vi "Set Shifter.vi"(8 "error in (no error)":errorcluster, 11 "High Gear?":bool) -> (0 "error out":errorcluster)   [LabVIEW 2018]
uses:
  <vilib>/Rock Robotics/WPI/Solenoid/WPI_SolenoidValue.ctl
  Implementation/Is High Gear.vi
  <vilib>/Rock Robotics/WPI/Solenoid/WPI_SolenoidSetEnum.vi
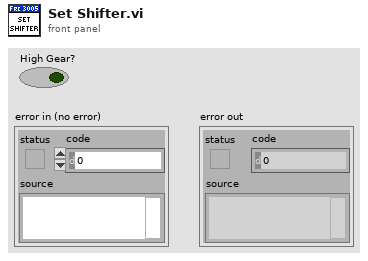
[diagram p1: front panel]
types:
  T1 = typedef "WPI_SolenoidValue.ctl" = enum16{"Off", "On", "Forward", "Reverse"}
  T2 = typedef "SPARKMAX6Motor.ctl" = cluster{"FrontLeftMaster":T3, "FrontLeftSlave1":T3, "FrontLeftSlave2":T3, "FrontRightMaster":T3, "FrontRightSlave1":T3, "FrontRightSlave2":T3}
  T3 = typedef "WPI_MotorControlDeviceRef.ctl" = cluster{"DeviceStatus":errorcluster, "Type":T4, "PWM":cluster{"PWM Channel":T5, "DeadBand":T6}, "CAN":cluster{"Device Number":u8, "SetOutput VI Ref":variant, "GetOutput VI Ref":variant, "Enable VI Ref":variant, "Disable VI Ref":variant, "Data":variant}, "Invert":bool, "DIO PWM":cluster{"PWM \"Enable\" Channel":T5, "DIOChannel":T7, "PWM Rate":dbl}}
  T4 = typedef "WPI_MotorControlType.ctl" = enum16{"PWM", "CAN", "DIO PWM"}
  T5 = typedef "FPGA_DIOPWMChannel.ctl" = enum8{"PWM 0", "PWM 1", "PWM 2", "PWM 3", "PWM 4", "PWM 5", "PWM 6", "PWM 7", "PWM 8", "PWM 9", "PWM MXP 0", "PWM MXP 1", "PWM MXP 2", "PWM MXP 3", "PWM MXP 4", "PWM MXP 5", "PWM MXP 6", "PWM MXP 7", "PWM MXP 8", "PWM MXP 9", "Invalid"}
  T6 = typedef "WPI_PWMDeadband.ctl" = cluster{"Name":string, "maxPositivePwm":i32, "minPositivePwm":i32, "centerPwm":i32, "maxNegativePwm":i32, "minNegativePwm":i32, "angularRange":u16}
  T7 = typedef "FPGA_DIOChannel.ctl" = enum8{"DIO 0", "DIO 1", "DIO 2", "DIO 3", "DIO 4", "DIO 5", "DIO 6", "DIO 7", "DIO 8", "DIO 9", "DIO MXP 0", "DIO MXP 1", "DIO MXP 2", "DIO MXP 3", "DIO MXP 4", "DIO MXP 5", "DIO MXP 6", "DIO MXP 7", "DIO MXP 8", "DIO MXP 9", "DIO MXP 10", "DIO MXP 11", "DIO MXP 12", "DIO MXP 13", "DIO MXP 14", "DIO MXP 15", "SPI Port CS1", "SPI Port CS2", "SPI Port CS3", "SPI Port MISO", "SPI Port MOSI", "Invalid"}
  T8 = typedef "WPI_SolenoidDevRef.ctl" = cluster{"DevStatus":errorcluster, "Pneumatics Control Module":u8, "Forward Solenoid Channel":T9, "Reverse Solenoid Channel":T9}
  T9 = typedef "WPI_SolenoidChannel.ctl" = enum8{"Solenoid 0", "Solenoid 1", "Solenoid 2", "Solenoid 3", "Solenoid 4", "Solenoid 5", "Solenoid 6", "Solenoid 7", "Invalid"}
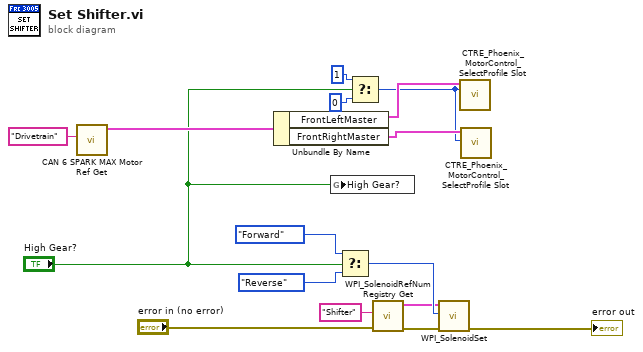
[diagram p0: block diagram]
diagram:
  n1 = call "CAN 6 SPARK MAX Motor Ref Get.vi"("refnum name"="Drivetrain") -> ("TalonSRX6MotorRef out"=w7:T2)  [unwired: 9 in, 1 out]
  n2 = Unbundle By Name(w7) -> ("FrontLeftMaster"=w6:T3, "FrontRightMaster"=w3:T3)
  n3 = global write "Is High Gear.vi" "High Gear?"("High Gear?") -> ()
  n4 = Select(t=WPI_SolenoidValue."Forward" ("Value"), s="High Gear?", f=WPI_SolenoidValue."Reverse" ("Value")) -> (s? t:f=w14:T1)
  n5 = Select(t=1 ("slotIdx"), s="High Gear?", f=0 ("slotIdx")) -> (s? t:f=w2:i32)
  n6 = call <vilib>:"WPI_SolenoidRefNum Registry Get.vi"("error in (no error)"="error in (no error)", "refnum name"="Shifter") -> ("error out"=w11:errorcluster, "SolenoidDevRef"=w10:T8)  [unwired: 8 in]
  n7 = call-poly <vilib>:"WPI_SolenoidSet.vi"("error in (no error)"=w11, "Value"=w14, "SolenoidDevRef"=w10) -> ("error out"=→"error out":errorcluster)  [unwired: 7 in, 1 out]
  n8 = call <vilib>:"CTRE_Phoenix_MotorControl_SelectProfile Slot.vi"("slotIdx"=w2, "PhoenixMotorControlDevRef"=w6) -> ()  [unwired: 8 in, 2 out]
  n9 = call <vilib>:"CTRE_Phoenix_MotorControl_SelectProfile Slot.vi"("slotIdx"=w2, "PhoenixMotorControlDevRef"=w3) -> ()  [unwired: 8 in, 2 out]
